vi "DSF.Engine.Memory.Cache.Plugin.Set Plugin Configuration.vi"(8 "error in (no error)":errorcluster, 10 "Plugin Configuration":refnum<class "DSF.Shared.Configuration.Plugin.lvclass">, 11 "Plugin Cache in":refnum<class "DSF.Engine.Memory.Cache.Plugin.lvclass">) -> (0 "error out":errorcluster, 3 "Plugin Cache out":refnum<class "DSF.Engine.Memory.Cache.Plugin.lvclass">)   [LabVIEW 2017, in "DSF.Engine.lvlib" / "DSF.Engine.Memory.Cache.Plugin.lvclass"]
uses:
  DSF.Engine.Memory.Cache.Plugin.lvclass
  Shared/Classes/Plugin/DSF.Shared.Configuration.Plugin.lvclass
  DSF.Engine.Memory.Cache.Plugin.lvclass/DSF.Engine.Memory.Cache.Plugin.ctl
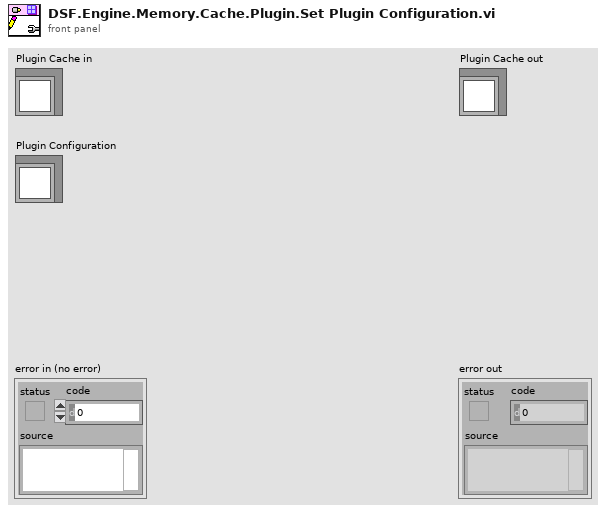
[diagram p1: front panel]
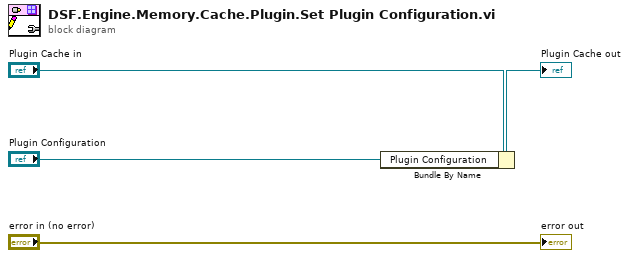
[diagram p0: block diagram]
diagram:
  n1 = Bundle By Name(cluster="Plugin Cache in", "Plugin Configuration"="Plugin Configuration") -> (→"Plugin Cache out":refnum<class "DSF.Engine.Memory.Cache.Plugin.lvclass">)
  "error out" <- "error in (no error)"
